vi "Write Waveform.vi"(8 "error in (no error)":errorcluster, 10 "Waveform":waveform(dbl)[](array[waveform]), 11 "Waveform_Task in":refnum<class "Waveform_Task.lvclass">) -> (0 "error out":errorcluster, 3 "Waveform_Task out":refnum<class "Waveform_Task.lvclass">)   [LabVIEW 2025, in "Waveform_Task.lvlib" / "Waveform_Task.lvclass"]
uses:
  Waveform_Task.lvclass
  Waveform_Task.lvclass/Waveform_Task.ctl
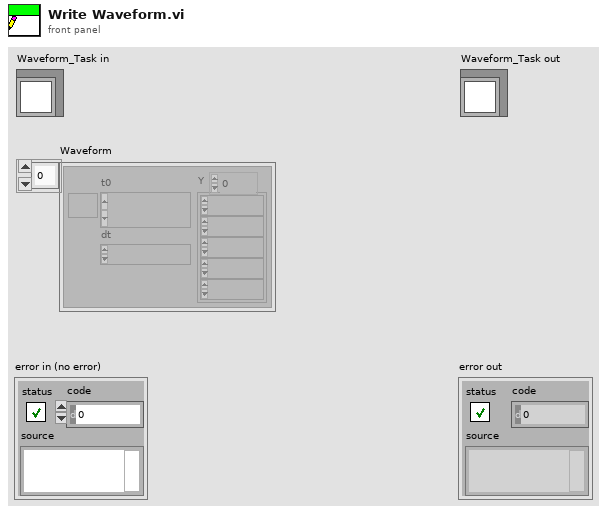
[diagram p1: front panel]
types:
  T1 = typedef "Task_Abstr.lvlib/Task_Abstr.lvclass/DataContainer.ctl" = map{string, T2}
  T2 = typedef "Task_Abstr.lvlib/Task_Abstr.lvclass/WaveformData.ctl" = cluster{"StartTime":timestamp, "StopTime":timestamp, "Waveform":waveform(dbl)[]}
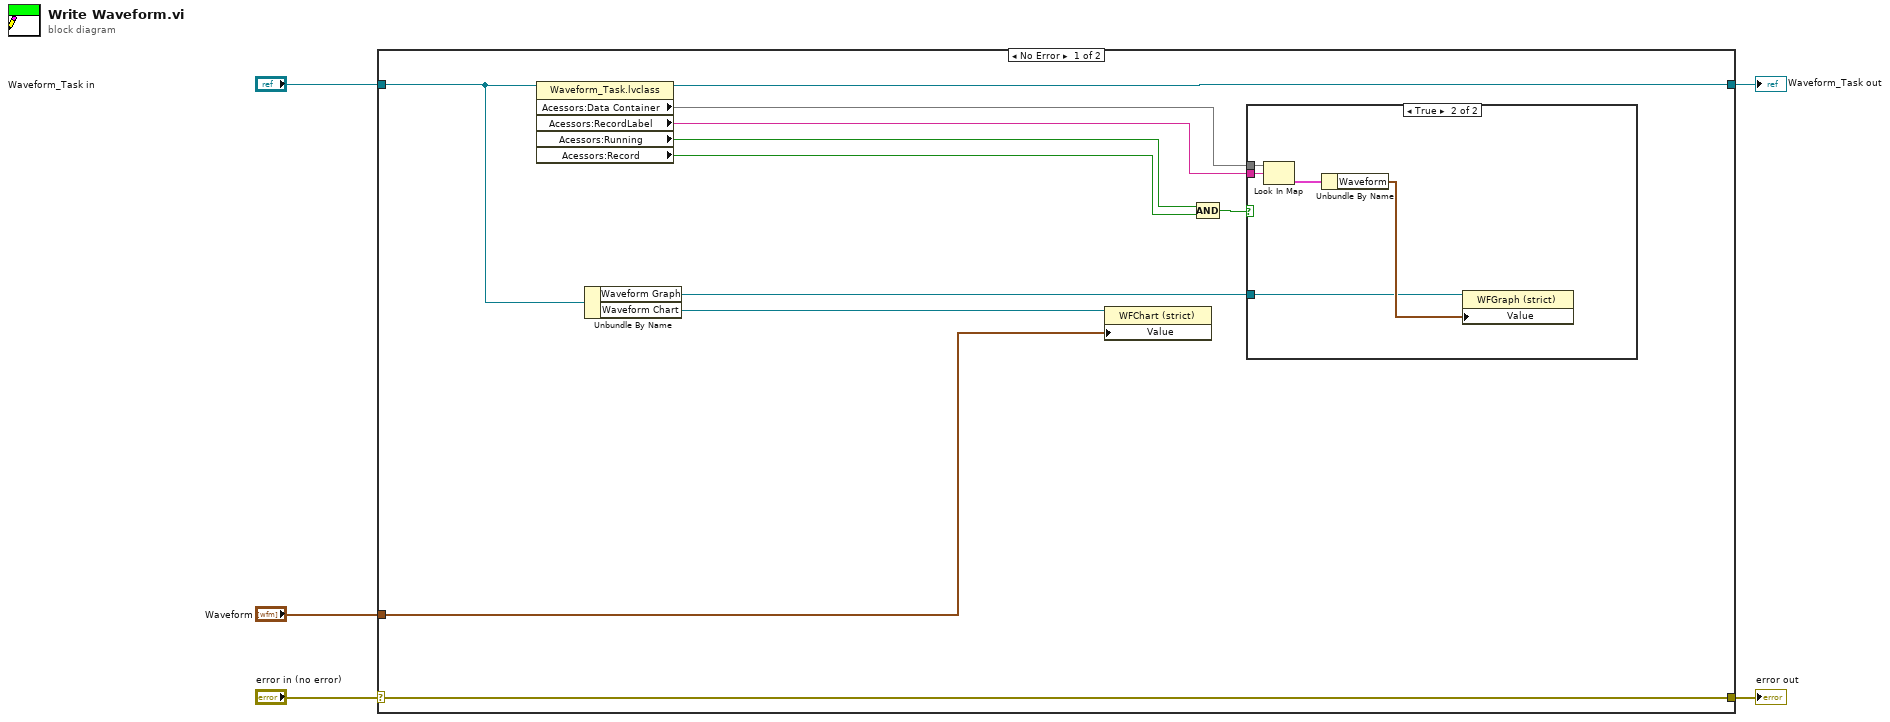
[diagram p0: block diagram]
diagram:
  n1 = case shown="No Error" "error in (no error)" {
    selector: "error in (no error)" -> [w16 w22]
    tunnel: [w16 w22] -> w4
    tunnel: [w7 w23] -> w2
    tunnel: "Waveform_Task in" -> [w8 w23]
    tunnel: "Waveform" -> [w6 _]
    frame No Error {
      n2 = property class="Waveform_Task.lvclass"(reference=w8) -> (reference out=w7:refnum<class "Waveform_Task.lvclass">, "Acessors:Data Container"=w14:T1, "Acessors:RecordLabel"=w13:string, "Acessors:Running"=w11:bool, "Acessors:Record"=w10:bool)  [unwired: 1 in, 1 out]
      n3 = Unbundle By Name(w8) -> ("Waveform Graph"=w12:refnum<vi>, "Waveform Chart"=w15:refnum<vi>)
      n4 = property class="WFChart (strict)"(reference=w15, "Value"=w6) -> ()  [unwired: 1 in, 2 out]
      n5 = Compound Arithmetic op=AND(w11, w10) -> (w9:bool)
      n6 = case shown="True" w9 {
        tunnel: w14 -> [_ w21]
        tunnel: w13 -> [_ w20]
        tunnel: w12 -> [_ w17]
        frame False {
        }
        frame True {
          n7 = Look In Map(map=w21, key=w20) -> (value=w19:T2)  [unwired: 1 in, 1 out]
          n8 = Unbundle By Name(w19) -> ("Waveform"=w18:waveform(dbl)[])
          n9 = property class="WFGraph (strict)"(reference=w17, "Value"=w18) -> ()  [unwired: 1 in, 2 out]
        }
      }
    }
    frame Error {
    }
  }
  "error out" <- w4
  "Waveform_Task out" <- w2
